vi "GetCurvesParams.vi"(8 "error in (no error)":errorcluster caption="entrée d'erreur (pas d'erreur)", 9 "CurvIndex":i32, 11 "Interface en entrée":refnum<class "Interface.lvclass"> caption="DNL_LabVIEW Object in") -> (0 "error out":errorcluster caption="sortie d'erreur", 2 "CurvePar Out":T1={"CurveName"="", "YParam"="", "XParam"="", "ZParam "="", "GroupName"="", "LinWdth"=1, "PntCol"=4294967295, "LinCol"=4294967295, "LablFor"=0, "XScale"=0, "YScale"=0, "Interpol"=2, "DisplayName"="", "FillType"=-1, "LineStyle"=0, "PntStyle"=12, "BarTyp"=0, "GraphIndex"=0, "Visible"=TRUE, "XScaleName"="", "YScaleName"="", "XYGraph_Ref"=refnum, "Data Only"=FALSE, "DataQ Ref"=refnum, "XParQ Ref"=refnum, "XParamInd"=0, "ScanInd"=0, "File Path"=path ""}, 3 "Interface en sortie":refnum<class "Interface.lvclass"> caption="DNL_LabVIEW Object out")   [LabVIEW 2019, in "Interface.lvclass"]
uses:
  Interface.lvclass
  CurveSetup.ctl
  Interface.lvclass/Interface.ctl
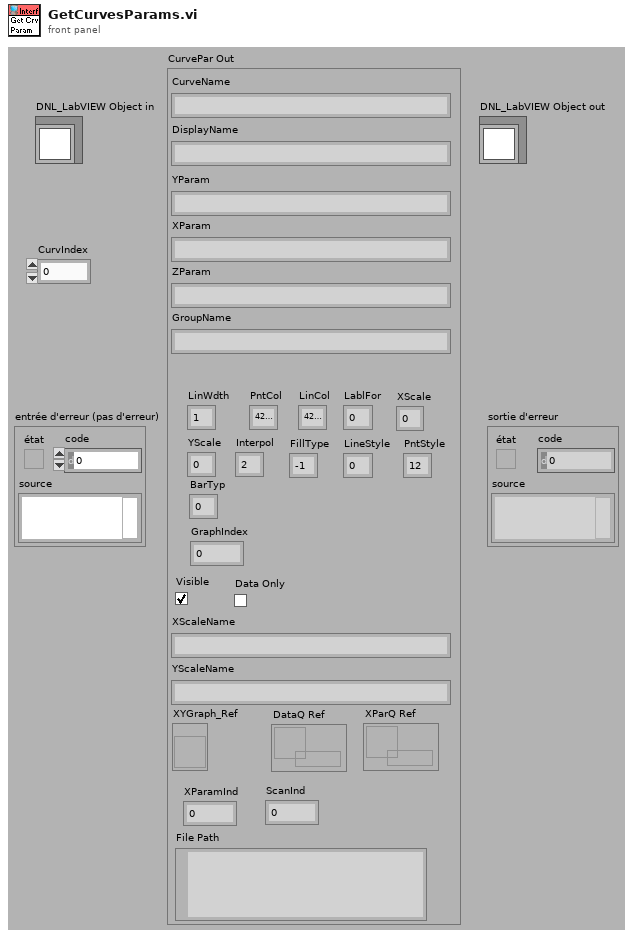
[diagram p1: front panel]
types:
  T1 = typedef "Interface.lvclass/CurveSetup.ctl" = cluster{"CurveName":string, "YParam":string, "XParam":string, "ZParam ":string, "GroupName":string, "LinWdth":u8, "PntCol":u32, "LinCol":u32, "LablFor":u8, "XScale":u32, "YScale":u32, "Interpol":u8, "DisplayName":string, "FillType":i16, "LineStyle":u8, "PntStyle":u8, "BarTyp":u8, "GraphIndex":i32, "Visible":bool, "XScaleName":string, "YScaleName":string, "XYGraph_Ref":refnum<vi>, "Data Only":bool, "DataQ Ref":refnum<queue>, "XParQ Ref":refnum<queue>, "XParamInd":i32, "ScanInd":i32, "File Path":path}
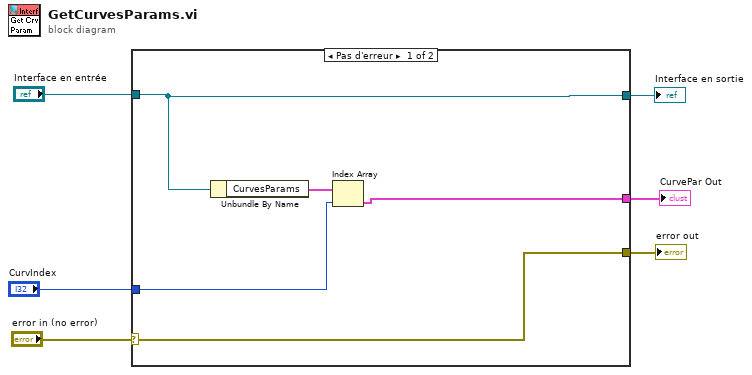
[diagram p0: block diagram]
diagram:
  n1 = case shown="Pas d'erreur" "error in (no error)" {
    selector: "error in (no error)" -> [w9 w13]
    tunnel: [w9 w13] -> w5
    tunnel: [w10 w12] -> w3
    tunnel: "Interface en entrée" -> [w10 w12]
    tunnel: "CurvIndex" -> [w11 _]
    tunnel: [w8 _] -> w1
    frame No Error {
      n2 = Unbundle By Name(w10) -> ("CurvesParams"=w7:T1[])
      n3 = Index Array(array=w7, index=w11) -> (element=w8:T1)
    }
    frame Error {
    }
  }
  "error out" <- w5
  "Interface en sortie" <- w3
  "CurvePar Out" <- w1
